vi "State Machine Kernel.vi"(4 "Init?":bool, 5 "Inputs":T3, 6 "StateData":T1) -> (0 "Terminated?":bool, 1 "Outputs":T2, 2 "StateData":T1)   [LabVIEW 2017]
uses:
  Controls/Outputs.ctl
  Controls/Inputs.ctl
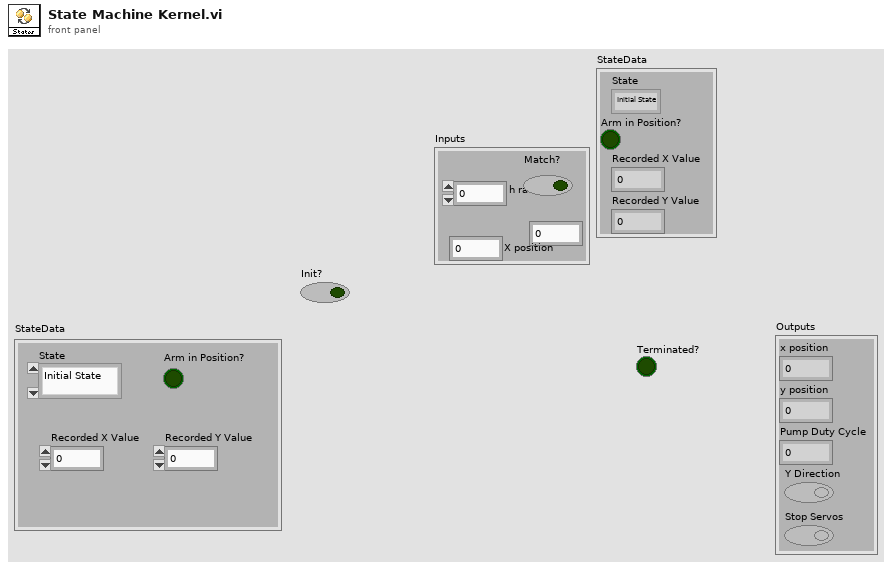
[diagram p1: front panel]
types:
  T1 = cluster{"State":enum16{"Initial State", "Pre Move", "Move Arm", "Fill Water"}, "Arm in Position?":bool, "Recorded X Value":dbl, "Recorded Y Value":dbl}
  T2 = typedef "Outputs.ctl" = cluster{"x position":dbl, "y position":dbl, "Pump Duty Cycle":dbl, "Y Direction":bool, "Stop Servos":bool}
  T3 = typedef "Inputs.ctl" = cluster{"X position":dbl, "Y position":dbl, "h ratio":dbl, "Match?":bool}
  T4 = enum16{"Initial State", "Pre Move", "Move Arm", "Fill Water"}
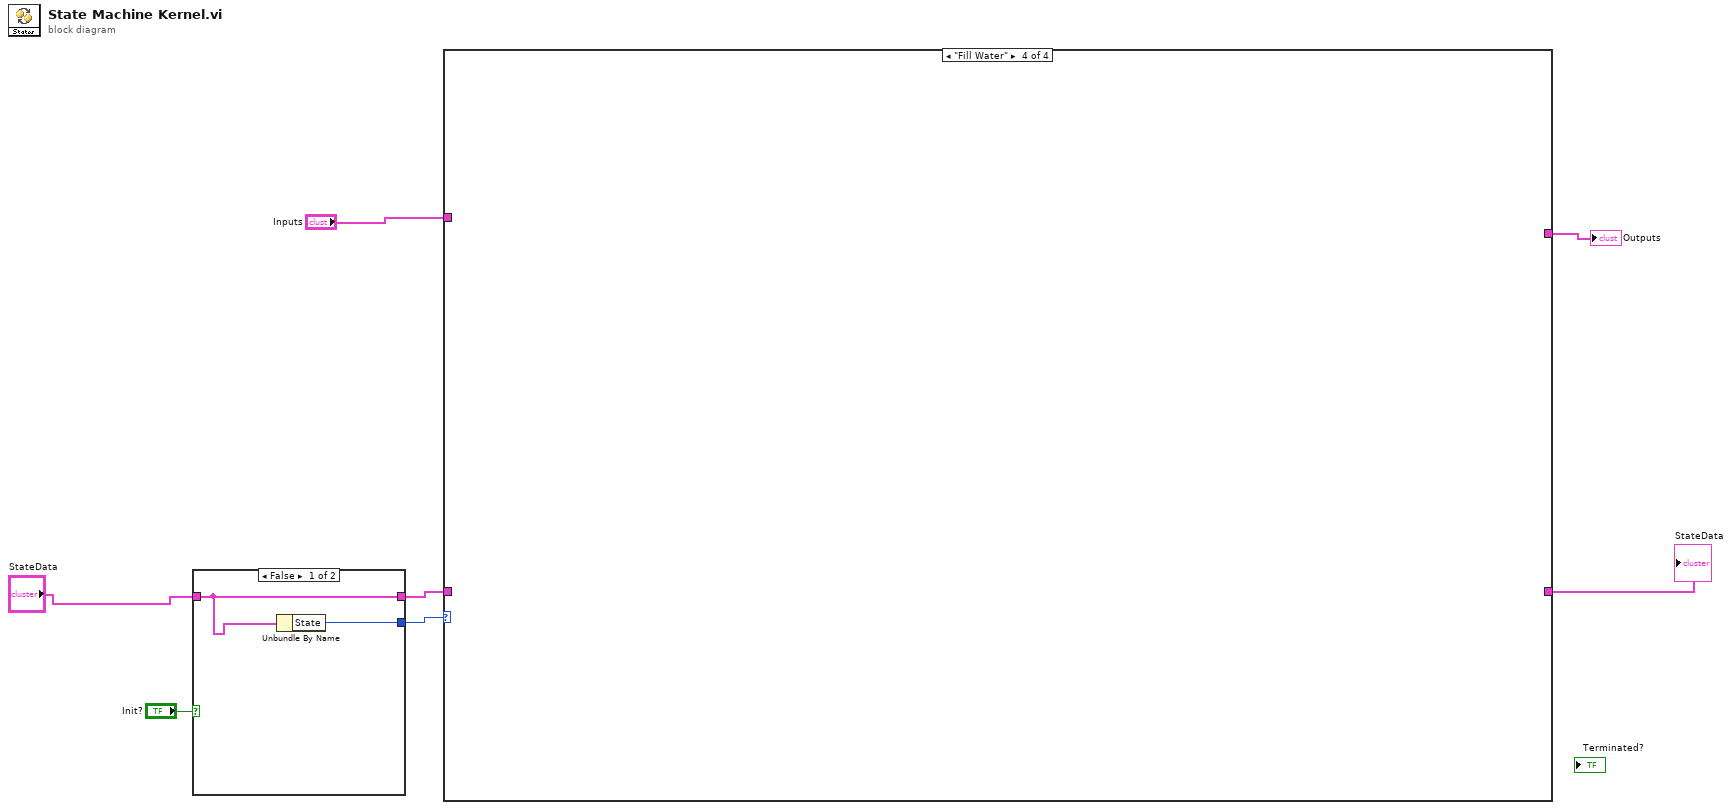
[diagram p0: block diagram]
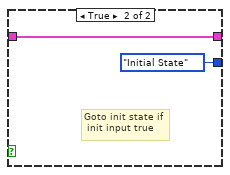
[diagram p2: hidden frame]
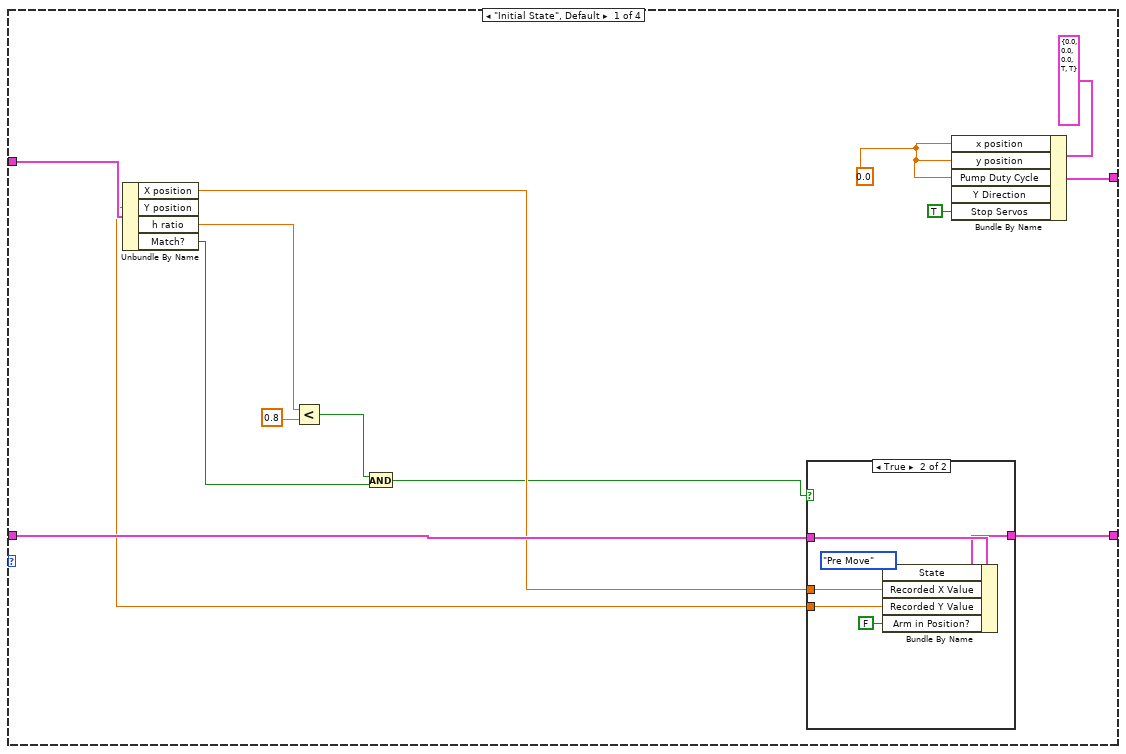
[diagram p3: hidden frame]
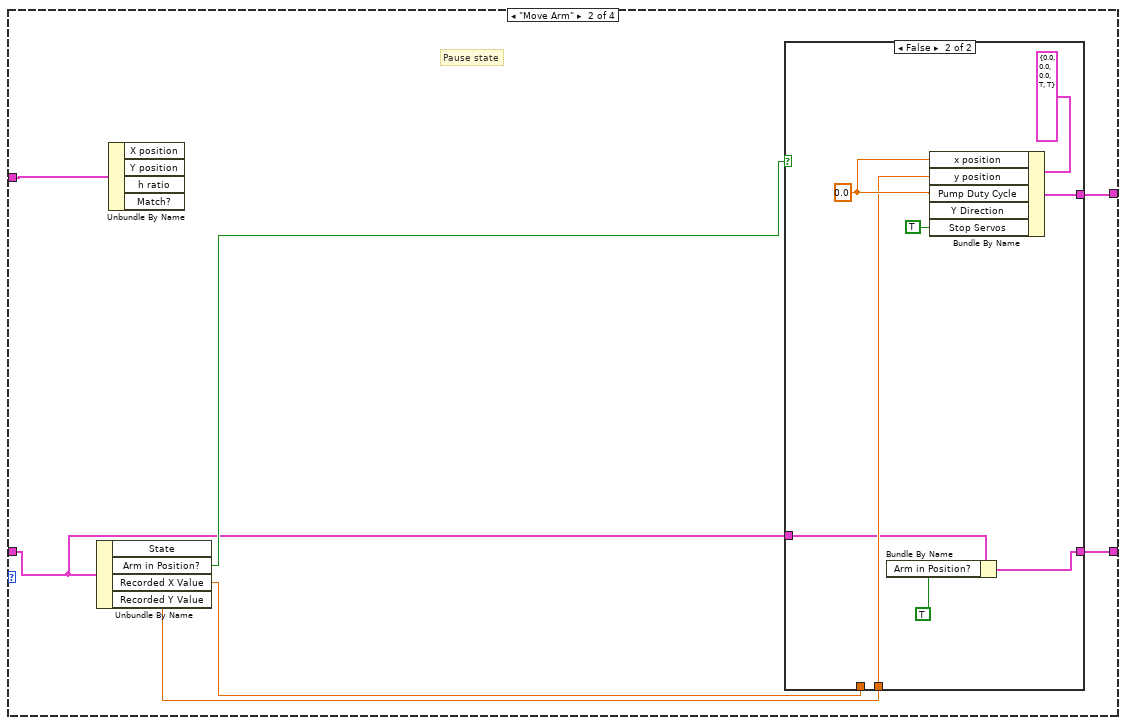
[diagram p5: hidden frame]
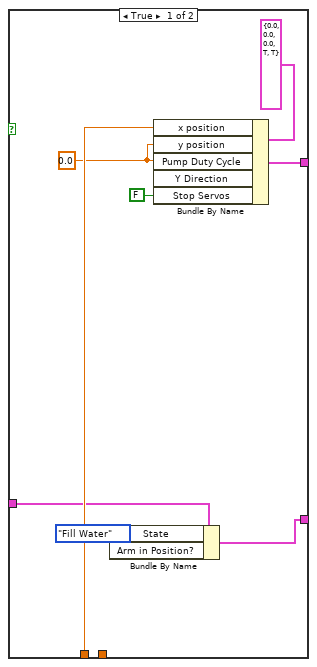
[diagram p6: hidden frame]
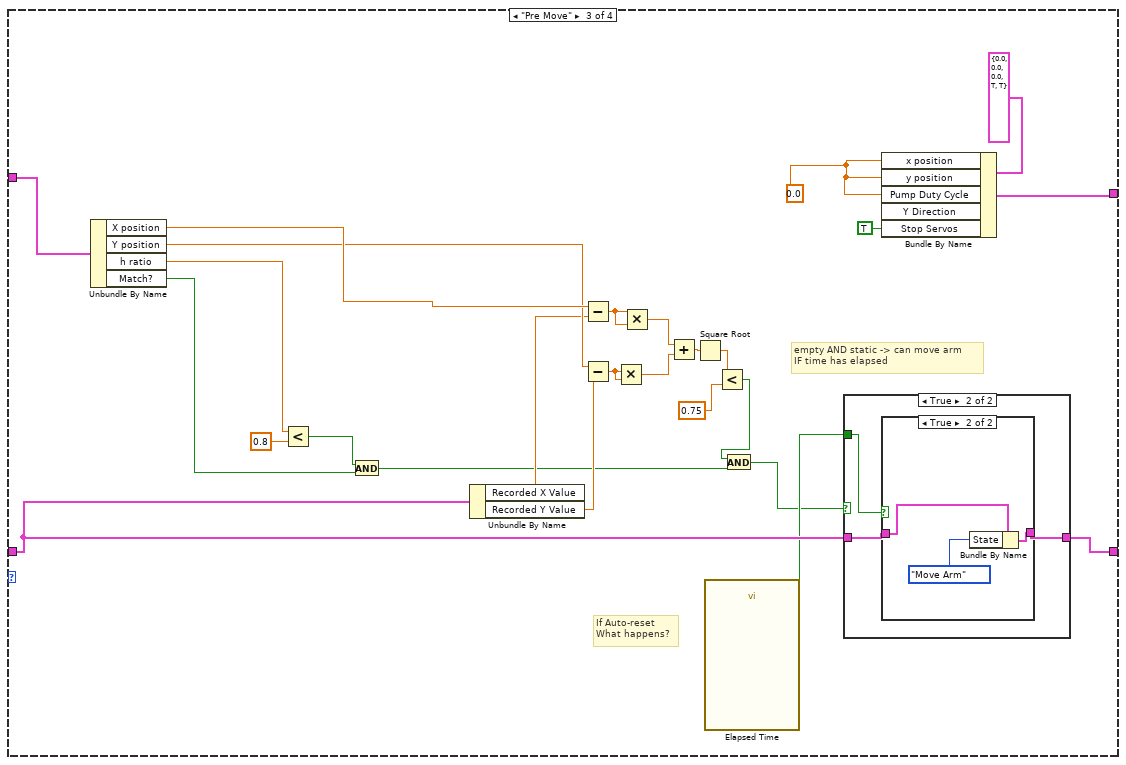
[diagram p7: hidden frame]
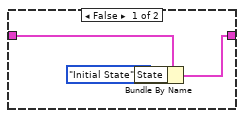
[diagram p8: hidden frame]
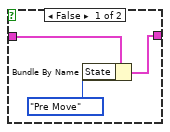
[diagram p9: hidden frame]
diagram:
  n1 = case shown="False" "Init?" {
    tunnel: "StateData" -> [w9 w11]
    tunnel: [w9 w11] -> w4
    tunnel: [w8 T4."Initial State" ("State")] -> w1
    frame False {
      n2 = Unbundle By Name(w9) -> ("State"=w8:T4)
    }
    frame True {
      # "Goto init state if\n init input true"
    }
  }
  n3 = case shown="\"Fill Water\"" w1 {
    tunnel: "Inputs" -> [w25 w38 w81 _]
    tunnel: [w21 w39 w63 _] -> w5
    tunnel: w4 -> [w19 w34 w79 _]
    tunnel: [w20 w33 w80 _] -> w3
    frame "Initial State", Default {
      w23 = 0.0
      n4 = Unbundle By Name(w25) -> ("X position"=w18:dbl, "Y position"=w17:dbl, "h ratio"=w13:dbl, "Match?"=w16:bool)
      n5 = Less?(x=w13, y=0.8) -> (x < y?=w12:bool)
      n6 = And(x=w12, y=w16) -> (x .and. y?=w15:bool)
      n7 = case shown="True" w15 {
        tunnel: w19 -> [w26 w32]
        tunnel: [w26 w31] -> w20
        tunnel: w18 -> [_ w29]
        tunnel: w17 -> [_ w28]
        frame False {
        }
        frame True {
          n8 = Bundle By Name(cluster=w32, "State"=T4."Pre Move", "Recorded X Value"=w29, "Recorded Y Value"=w28, "Arm in Position?"=FALSE) -> (w31:T1)
        }
      }
      n9 = Bundle By Name(cluster=T2 {"x position"=0.0, "y position"=0.0, "Pump Duty Cycle"=0.0, "Y Direction"=TRUE, "Stop Servos"=TRUE} ("Outputs"), "x position"=w23, "y position"=w23, "Pump Duty Cycle"=w23, "Stop Servos"=TRUE) -> (w21:T2)  [unwired: 1 in]
    }
    frame "Move Arm" {
      # "Pause state"
      n10 = Unbundle By Name(w34) -> ("Arm in Position?"=w37:bool, "Recorded X Value"=w36:dbl, "Recorded Y Value"=w35:dbl)  [unwired: 1 out]
      n11 = Unbundle By Name(w38) -> ()  [unwired: 4 out]
      n12 = case shown="False" w37 {
        tunnel: [w45 w53] -> w39
        tunnel: w36 -> [w44 _]
        tunnel: w35 -> [_ w51]
        tunnel: w34 -> [w42 w50]
        tunnel: [w41 w49] -> w33
        frame True {
          w43 = 0.0
          n13 = Bundle By Name(cluster=w42, "State"=T4."Fill Water") -> (w41:T1)  [unwired: 1 in]
          n14 = Bundle By Name(cluster=T2 {"x position"=0.0, "y position"=0.0, "Pump Duty Cycle"=0.0, "Y Direction"=TRUE, "Stop Servos"=TRUE} ("Outputs"), "x position"=w44, "y position"=w43, "Pump Duty Cycle"=w43, "Stop Servos"=FALSE) -> (w45:T2)  [unwired: 1 in]
        }
        frame False {
          w52 = 0.0
          n15 = Bundle By Name(cluster=w50, "Arm in Position?"=TRUE) -> (w49:T1)
          n16 = Bundle By Name(cluster=T2 {"x position"=0.0, "y position"=0.0, "Pump Duty Cycle"=0.0, "Y Direction"=TRUE, "Stop Servos"=TRUE} ("Outputs"), "x position"=w52, "y position"=w51, "Pump Duty Cycle"=w52, "Stop Servos"=TRUE) -> (w53:T2)  [unwired: 1 in]
        }
      }
    }
    frame "Pre Move" {
      w65 = 0.0
      # "empty AND static -> can move arm\nIF time has elapsed"
      # "If Auto-reset\nWhat happens?"
      n17 = Unbundle By Name(w81) -> ("X position"=w78:dbl, "Y position"=w77:dbl, "h ratio"=w59:dbl, "Match?"=w60:bool)
      n18 = Less?(x=w59, y=0.8) -> (x < y?=w61:bool)
      n19 = And(x=w61, y=w60) -> (x .and. y?=w58:bool)
      n20 = Unbundle By Name(w79) -> ("Recorded X Value"=w76:dbl, "Recorded Y Value"=w75:dbl)
      n21 = Subtract(x=w78, y=w76) -> (x-y=w74:dbl)
      n22 = Subtract(x=w77, y=w75) -> (x-y=w73:dbl)
      n23 = Multiply(x=w73, y=w73) -> (x*y=w71:dbl)
      n24 = Multiply(x=w74, y=w74) -> (x*y=w72:dbl)
      n25 = Add(x=w72, y=w71) -> (x+y=w70:dbl)
      n26 = Square Root(x=w70) -> (sqrt(x)=w68:dbl)
      n27 = call "Elapsed Time"() -> ("Time has Elapsed"=w67:bool)  [unwired: 12 in, 7 out]
      n28 = Less?(x=w68, y=0.75) -> (x < y?=w57:bool)
      n29 = And(x=w57, y=w58) -> (x .and. y?=w56:bool)
      n30 = case shown="True" w56 {
        tunnel: w79 -> [w84 w87]
        tunnel: [w83 w85] -> w80
        tunnel: w67 -> [_ w86]
        frame False {
          n31 = Bundle By Name(cluster=w84, "State"=T4."Initial State") -> (w83:T1)
        }
        frame True {
          n32 = case shown="True" w86 {
            tunnel: w87 -> [w89 w92]
            tunnel: [w88 w91] -> w85
            frame False {
              n33 = Bundle By Name(cluster=w89, "State"=T4."Pre Move") -> (w88:T1)
            }
            frame True {
              n34 = Bundle By Name(cluster=w92, "State"=T4."Move Arm") -> (w91:T1)
            }
          }
        }
      }
      n35 = Bundle By Name(cluster=T2 {"x position"=0.0, "y position"=0.0, "Pump Duty Cycle"=0.0, "Y Direction"=TRUE, "Stop Servos"=TRUE} ("Outputs"), "x position"=w65, "y position"=w65, "Pump Duty Cycle"=w65, "Stop Servos"=TRUE) -> (w63:T2)  [unwired: 1 in]
    }
    frame "Fill Water" {
    }
  }
  "Outputs" <- w5
  "StateData" <- w3
